vi "RTC.vi"(11 "Data In":T1) -> (3 "Data Out":T1={"Port"="", "All Code"="Hi"})   [LabVIEW 2016]
uses:
  uPythonX/PythonData.ctl
  uPythonX/uPythonX.xctl
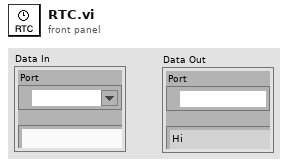
[diagram p1: front panel]
types:
  T1 = typedef "uPythonX.xctl/PythonData.ctl" = cluster{"Port":refnum<visa-resource-name>, "All Code":string}
  T2 = typedef "LVDateTimeRec.ctl" = cluster{"fractional second":dbl, "second":i32, "minute":i32, "hour":i32, "day of month":i32, "month":i32, "year":i32, "day of week":i32, "day of year":i32, "DST":i32}
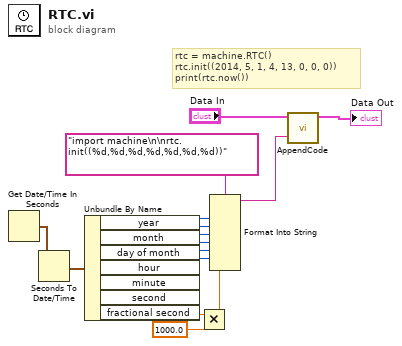
[diagram p0: block diagram]
diagram:
  # "rtc = machine.RTC()\nrtc.init((2014, 5, 1, 4, 13, 0, 0, 0))\nprint(rtc.now())"
  n1 = Get Date/Time In Seconds() -> (seconds since 1Jan1904=w11:timestamp)
  n2 = Seconds To Date/Time(time stamp (now)=w11) -> (date time rec=w10:T2)  [unwired: 1 in]
  n3 = Unbundle By Name(w10) -> ("year"=w9:i32, "month"=w8:i32, "day of month"=w7:i32, "hour"=w6:i32, "minute"=w5:i32, "second"=w4:i32, "fractional second"=w3:dbl)
  n4 = Multiply(x=w3, y=1000.0) -> (x*y=w1:dbl)
  n5 = Format Into String(format string="import machine\n\nrtc.init((%d,%d,%d,%d,%d,%d,%d))", w9, w8, w7, w6, w5, w4, w1) -> (resulting string=w12:string)  [unwired: 2 in, 1 out]
  n6 = call "AppendCode.vi"("New Code"=w12, "Data In"="Data In") -> ("Data Out"=→"Data Out":T1)  [unwired: 9 in]
